vi "Programa_robot_final_3.vi"() -> ()   [LabVIEW 2019]
uses:
  <vilib>/Instr/_visa.llb/VISA Configure Serial Port (Instr).vi
  Global_STOP.vi
  <vilib>/regexp/Match Regular Expression.xnode
panel:
  in  "STOP TEST 3":bool
  in  "stop socket 4":bool
  in  "Abrir socket 2":bool
  in  "Cerrar socket 2":bool
  in  "Interruptor Error 2":bool
  in  "stop 4":bool
  in  "stop 3":bool
  in  "stop 2":bool
  in  "stop socket 3":bool
  out "Datos_QR":string
  in  "Interruptor Error":bool
  in  "Cerrar socket":bool
  in  "Abrir socket":bool
  out "Error_QR":bool
  out "return count":u32
  out "lectura puerto serie":u32
  out "dato escrito puerto serie":string
  out "OK, Fault 2":bool
  out "error out":errorcluster {"code" format="%f"}
  in  "STOP TEST 2":bool
  out "Datos_QR 2":string
  out "NUMERO ASICS TESTEADOS":i32
  out ".not. x?":bool
  in  "Config File":path=path "C:/Trabajo_Robot/Test Asic Javi_2021/Origen Socket SERVO_PCB_BUENO_v5 (muchos asics)/CONFIG/configuracion_robot_CTAV2022A.test"
  in  "SELECCION DE TEST":string(combo)
  in  "?":bool
  out "Boolean":bool
  in  "stop socket 2":bool
  out "Bytes at port 3":u32=1
  in  "IN y":string(combo)="00"
  in  "IN x":string(combo)="00"
  in  "NOK y":string(combo)="00"
  in  "NOK x":string(combo)="00"
  in  "OK y":string(combo)="00"
  in  "OK x":string(combo)="00"
  in  "Operator's name":string(combo)="Juan Rodríguez"
  in  "?":bool
  in  "Fichero de registro":path=path "C:/Trabajo_Robot/Pruebas/Pruebas.txt"
  in  "Path Out Report":path=path "C:/Trabajo_Robot/desde Marzo 2023/Pruebas_PC_APD/RESULT_TEST_C_LABP0/Test_33_ASIC_Referencia"
  in  "stop socket":bool
  out "Bytes at port 1":u32
  out "Iteraciones":i32
  out "Lectura buffer":string="1"
  in  "Delay (ms)":dbl=1.0 min=1.0 max=9.0 step=1.0
  out "Bytes at port 2":u32=1
  in  "Interruptor":bool=TRUE
  in  "stop":bool
  # "SI SE PRESIONA EL BOTON STOP PARA DETENER EL TEST,\nHAY QUE APAGAR Y VOLVER A ENCENDER EL ARDUINO"
  # "x: columna en cada bandeja \ny: fila en cada bandeja"
  # "Funcionamiento: en la primera iteración, el efector se desplaza desde el origen hasta la celda\nintroducida, hace una pausa, va a la posición del socket (0,0), hace otra pausa, va a la celda\nde salida y vuelve al origen. En las iteraciones siguientes hará lo mismo pero recorriendo las\nceldas de la bandeja sucesivamente. Que el desplazamiento se produzca hacia una celda de\nla bandeja OK o de la bandeja NOK depende de la salidad del programa de test de Asics."
types:
  T1 = enum16{"open", "replace", "create", "open or create", "replace or create", "replace or create with confirmation"}
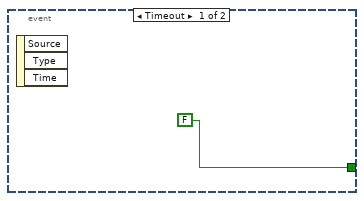
[diagram p2: hidden frame]
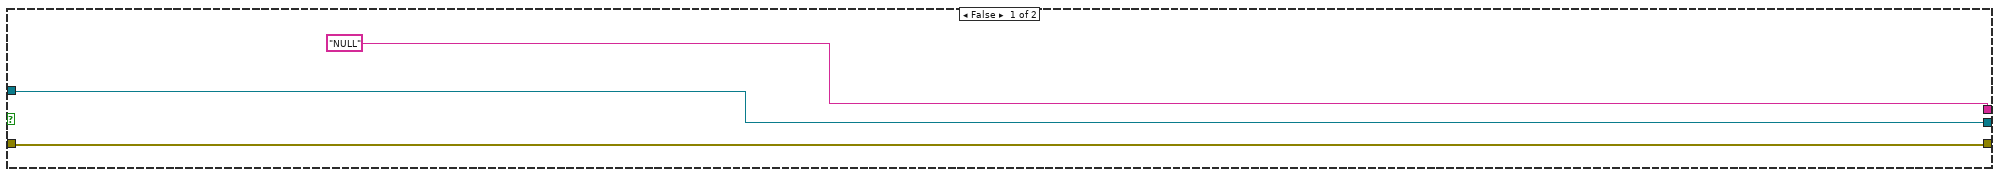
[diagram p5: hidden frame]
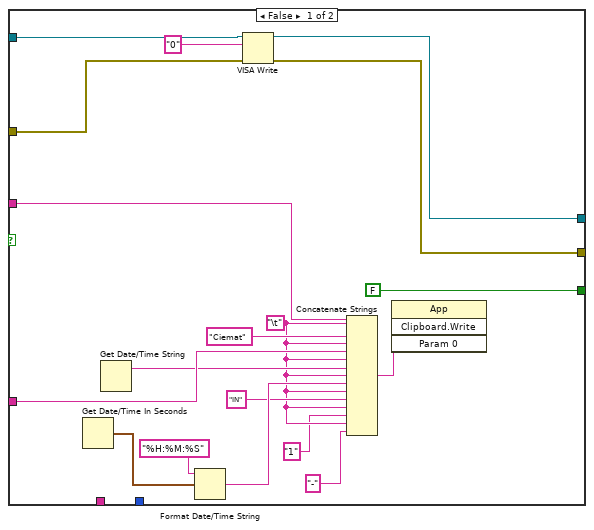
[diagram p7: hidden frame]
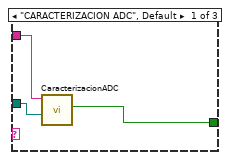
[diagram p8: hidden frame]
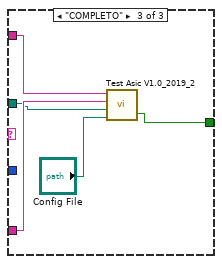
[diagram p9: hidden frame]
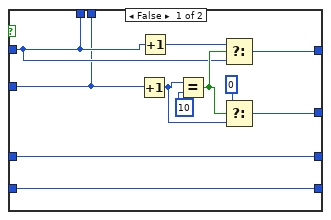
[diagram p11: hidden frame]
diagram:
  n1 = control-ref of="stop 2"() -> ()  [unwired: 1 out]
  n2 = control-ref of="stop 3"() -> ()  [unwired: 1 out]
  n3 = control-ref of="stop socket 3"() -> ()  [unwired: 1 out]
  n4 = control-ref of="Cerrar socket"() -> (w11:refnum<vi>)
  n5 = control-ref of="stop socket"() -> (w10:refnum<vi>)
  n6 = control-ref of="STOP TEST 2"() -> (w8:refnum<vi>)
  n7 = control-ref of="Abrir socket"() -> (w7:refnum<vi>)
  n8 = control-ref of="stop"() -> (w9:refnum<vi>)
  n9 = control-ref of="Interruptor Error"() -> (w12:refnum<vi>)
  n10 = property class="Bool (strict)"(reference=w8, "Visible"=FALSE) -> ()  [unwired: 1 in, 2 out]
  n11 = property class="Bool (strict)"(reference=w7, "Visible"=FALSE) -> ()  [unwired: 1 in, 2 out]
  n12 = property class="Bool (strict)"(reference=w12, "Visible"=FALSE) -> ()  [unwired: 1 in, 2 out]
  n13 = property class="Bool (strict)"(reference=w11, "Visible"=FALSE) -> ()  [unwired: 1 in, 2 out]
  n14 = property on="Boolean" class="Bool (strict)"("Visible"=FALSE) -> ()  [unwired: 2 in, 2 out]
  n15 = property class="Bool"(reference=w10, "Visible"=FALSE) -> ()  [unwired: 1 in, 2 out]
  n16 = property class="Bool"(reference=w9, "Visible"=FALSE) -> ()  [unwired: 1 in, 2 out]
  n17 = flat-sequence {
    tunnel: [w54] -> w18
    tunnel: ["Fichero de registro"] -> w17
    tunnel: ["SELECCION DE TEST"] -> w16
    tunnel: ["NOK y"] -> w33
    tunnel: ["NOK x"] -> w32
    tunnel: ["OK y"] -> w31
    tunnel: ["OK x"] -> w30
    tunnel: ["IN y"] -> w29
    tunnel: ["IN x"] -> w28
    tunnel: [w57] -> w27
    tunnel: [w58] -> w26
    tunnel: ["IN y"] -> w25
    tunnel: ["IN x"] -> w24
    tunnel: w17 -> [w56]
    frame #0 {
      n18 = while {
        stop <- "?" stop-if-true
        n19 = Not(x="?") -> (.not. x?=w50:bool)
        "Boolean" <- w50
        n20 = property on="Boolean" class="Bool (strict)"("Blinking"=w50) -> ()  [unwired: 2 in, 2 out]
      }
      n21 = global write "Global_STOP.vi" "stop"(FALSE ("stop")) -> ()
    }
    frame #1 {
      n22 = Not(x="?") -> (.not. x?=w54:bool)
      ".not. x?" <- w54
    }
    frame #2 {
      n23 = Open/Create/Replace File(file path (use dialog)=w56, operation (0:open)=T1."open", access (0:read/write)=enum16{"read/write", "read-only", "write-only"}."write-only") -> (refnum out=w69:refnum<file>, error out=w71:errorcluster)  [unwired: 3 in, 1 out]
      n24 = Set File Position(refnum=w69, from (0:start)=enum16{"start", "end", "current"}."end", error in=w71) -> (refnum out=w70:refnum<file>, error out=w72:errorcluster)  [unwired: 1 in]
      n25 = Write to Text File(file (use dialog)=w70, text="\r\n", error in=w72) -> (refnum out=w58:refnum<file>, error out=w57:errorcluster)  [unwired: 1 in, 1 out]
    }
  }
  n26 = Decimal String To Number(string=w25) -> (number=w23:i32)  [unwired: 2 in, 1 out]
  n27 = Decimal String To Number(string=w24) -> (number=w20:i32)  [unwired: 2 in, 1 out]
  n28 = Multiply(x=10, y=w23) -> (x*y=w21:i32)
  n29 = Decimal String To Number(string=w31) -> (number=w35:i32)  [unwired: 2 in, 1 out]
  n30 = Decimal String To Number(string=w30) -> (number=w34:i32)  [unwired: 2 in, 1 out]
  n31 = Decimal String To Number(string=w33) -> (number=w37:i32)  [unwired: 2 in, 1 out]
  n32 = Decimal String To Number(string=w32) -> (number=w36:i32)  [unwired: 2 in, 1 out]
  n33 = call-poly "VISA Configure Serial Port"("VISA resource name"=refnum<visa-resource-name> "COM9", "baud rate (9600)"=u32 9600, "data bits (8)"=u16 8) -> ("VISA resource name out"=w41:refnum<visa-resource-name>, "error out"=w44:errorcluster)  [unwired: 11 in]
  n34 = Add(x=w21, y=w20) -> (x+y=w19:i32)
  n35 = while {
    shift-right: [w82] -> w42
    shift-left: w44 -> [w123]
    tunnel: w41 -> [w121]
    tunnel: [w84] -> w43
    tunnel: w26 -> [w114]
    tunnel: [w113] -> w40
    tunnel: w27 -> [w112]
    tunnel: [w111] -> w39
    tunnel: w28 -> [w109]
    tunnel: w29 -> [w108]
    tunnel: w30 -> [w107]
    tunnel: w31 -> [w106]
    tunnel: w32 -> [w105]
    tunnel: w33 -> [w104]
    shift-right: [w97] -> _
    shift-left: w37 -> [w103]
    shift-right: [w99] -> _
    shift-left: w36 -> [w102]
    shift-right: [w96] -> _
    shift-left: w35 -> [w101]
    shift-right: [w98] -> _
    shift-left: w34 -> [w100]
    tunnel: w19 -> [w95]
    tunnel: w18 -> [w87]
    tunnel: w16 -> [w86]
    tunnel: [w80] -> w14
    i -> [w85]
    stop <- w80 stop-if-true
    n36 = flat-sequence {
      tunnel: w123 -> [w176]
      tunnel: w121 -> [w165]
      tunnel: [w167] -> w120
      tunnel: [w166] -> w119
      tunnel: w109 -> [w146]
      tunnel: w108 -> [w145]
      tunnel: w107 -> [w144]
      tunnel: w106 -> [w143]
      tunnel: w105 -> [w142]
      tunnel: w104 -> [w141]
      tunnel: w120 -> [w913]
      tunnel: w119 -> [w912]
      tunnel: [w911] -> w94
      tunnel: [w910] -> w92
      tunnel: [w909] -> _
      tunnel: w94 -> [w929]
      tunnel: [w927] -> w93
      tunnel: w92 -> [w928]
      tunnel: [w926] -> w91
      tunnel: w93 -> [w949]
      tunnel: w91 -> [w948]
      tunnel: w85 -> [w950]
      tunnel: [w946] -> w90
      tunnel: [w945] -> w89
      tunnel: [w944] -> w88
      tunnel: w85 -> [w1038]
      tunnel: [w1040] -> w117
      tunnel: [w1039] -> w116
      tunnel: [w1036] -> w110
      tunnel: w90 -> [w1035]
      tunnel: w89 -> [w1034]
      tunnel: w88 -> [w1033]
      tunnel: w87 -> [w1028]
      tunnel: w86 -> [w1031]
      tunnel: w85 -> [w1030]
      tunnel: [w1101] -> w115
      tunnel: [w1103] -> w118
      tunnel: w117 -> [w1102]
      tunnel: w116 -> [w1100]
      tunnel: w114 -> [w1107]
      tunnel: [w1106] -> w113
      tunnel: w112 -> [w1105]
      tunnel: [w1104] -> w111
      tunnel: w85 -> [w1097]
      tunnel: w110 -> [w1096]
      tunnel: w103 -> [w1092]
      tunnel: w102 -> [w1095]
      tunnel: w101 -> [w1094]
      tunnel: w100 -> [w1093]
      tunnel: [w1091] -> w97
      tunnel: [w1090] -> w99
      tunnel: [w1089] -> w96
      tunnel: [w1088] -> w98
      tunnel: w95 -> [w1087]
      tunnel: w85 -> [w1086]
      tunnel: [w1085] -> _
      frame #0 {
        n37 = for {
          N: 2 -> [_]
          shift-right: [w788] -> _
          shift-left: w146 -> [w793]
          shift-right: [w791] -> w162
          shift-left: w165 -> [w792]
          shift-right: [w789] -> w161
          shift-left: w176 -> [w790]
          n38 = xnode "Match Regular Expression"("input string"=w793, "regular expression"="-?\\d") -> ("whole match"=w787:string, "after match"=w788:string)  [unwired: 4 in, 3 out]
          n39 = VISA Write(VISA resource name=w792, write buffer=w787, error in (no error)=w790) -> (VISA resource name out=w791:refnum<visa-resource-name>, error out=w789:errorcluster)  [unwired: 1 out]
        }
        n40 = for {
          N: 2 -> [_]
          shift-right: [w666] -> _
          shift-left: w145 -> [w671]
          shift-right: [w669] -> w156
          shift-left: w162 -> [w670]
          shift-right: [w667] -> w155
          shift-left: w161 -> [w668]
          n41 = xnode "Match Regular Expression"("input string"=w671, "regular expression"="-?\\d") -> ("whole match"=w665:string, "after match"=w666:string)  [unwired: 4 in, 3 out]
          n42 = VISA Write(VISA resource name=w670, write buffer=w665, error in (no error)=w668) -> (VISA resource name out=w669:refnum<visa-resource-name>, error out=w667:errorcluster)  [unwired: 1 out]
        }
        n43 = for {
          N: 2 -> [_]
          shift-right: [w544] -> _
          shift-left: w144 -> [w549]
          shift-right: [w547] -> w158
          shift-left: w156 -> [w548]
          shift-right: [w545] -> w157
          shift-left: w155 -> [w546]
          n44 = xnode "Match Regular Expression"("input string"=w549, "regular expression"="-?\\d") -> ("whole match"=w543:string, "after match"=w544:string)  [unwired: 4 in, 3 out]
          n45 = VISA Write(VISA resource name=w548, write buffer=w543, error in (no error)=w546) -> (VISA resource name out=w547:refnum<visa-resource-name>, error out=w545:errorcluster)  [unwired: 1 out]
        }
        n46 = for {
          N: 2 -> [_]
          shift-right: [w422] -> _
          shift-left: w143 -> [w427]
          shift-right: [w425] -> w150
          shift-left: w158 -> [w426]
          shift-right: [w423] -> w149
          shift-left: w157 -> [w424]
          n47 = xnode "Match Regular Expression"("input string"=w427, "regular expression"="-?\\d") -> ("whole match"=w421:string, "after match"=w422:string)  [unwired: 4 in, 3 out]
          n48 = VISA Write(VISA resource name=w426, write buffer=w421, error in (no error)=w424) -> (VISA resource name out=w425:refnum<visa-resource-name>, error out=w423:errorcluster)  [unwired: 1 out]
        }
        n49 = for {
          N: 2 -> [_]
          shift-right: [w300] -> _
          shift-left: w142 -> [w305]
          shift-right: [w303] -> w152
          shift-left: w150 -> [w304]
          shift-right: [w301] -> w151
          shift-left: w149 -> [w302]
          n50 = xnode "Match Regular Expression"("input string"=w305, "regular expression"="-?\\d") -> ("whole match"=w299:string, "after match"=w300:string)  [unwired: 4 in, 3 out]
          n51 = VISA Write(VISA resource name=w304, write buffer=w299, error in (no error)=w302) -> (VISA resource name out=w303:refnum<visa-resource-name>, error out=w301:errorcluster)  [unwired: 1 out]
        }
        n52 = for {
          N: 2 -> [_]
          shift-right: [w178] -> _
          shift-left: w141 -> [w183]
          shift-right: [w181] -> w148
          shift-left: w152 -> [w182]
          shift-right: [w179] -> w147
          shift-left: w151 -> [w180]
          n53 = xnode "Match Regular Expression"("input string"=w183, "regular expression"="-?\\d") -> ("whole match"=w177:string, "after match"=w178:string)  [unwired: 4 in, 3 out]
          n54 = VISA Write(VISA resource name=w182, write buffer=w177, error in (no error)=w180) -> (VISA resource name out=w181:refnum<visa-resource-name>, error out=w179:errorcluster)  [unwired: 1 out]
        }
        n55 = Number To Decimal String(number="Delay (ms)") -> (decimal integer string=w170:string)  [unwired: 1 in]
        n56 = VISA Write(VISA resource name=w148, write buffer=w170, error in (no error)=w147) -> (VISA resource name out=w172:refnum<visa-resource-name>, error out=w171:errorcluster)  [unwired: 1 out]
        n57 = Select(t="1" ("write buffer"), s="Interruptor", f="0" ("write buffer")) -> (s? t:f=w168:string)
        n58 = VISA Write(VISA resource name=w172, write buffer=w168, error in (no error)=w171) -> (VISA resource name out=w167:refnum<visa-resource-name>, error out=w166:errorcluster)  [unwired: 1 out]
      }
      frame #1 {
        n59 = while {
          shift-right: [w919] -> w910
          shift-left: w912 -> [w924]
          tunnel: ["stop socket"] -> _
          shift-right: [w920] -> w911
          shift-left: w913 -> [w925]
          tunnel: ["stop socket"] -> w909
          stop <- w914 stop-if-true
          n60 = property class="Instr"(reference=w925, error in=w924) -> (reference out=w923:refnum<visa-resource-name>, error out=w922:errorcluster, "Bytes at Port"=w921:u32)
          "Bytes at port 1" <- w921
          n61 = VISA Read(VISA resource name=w923, byte count=w921, error in (no error)=w922) -> (VISA resource name out=w920:refnum<visa-resource-name>, read buffer=w918:string, error out=w919:errorcluster)  [unwired: 1 out]
          n62 = Equal?(x="2", y=w918) -> (x = y?=w916:bool)
          n63 = Or(x=w916, y="stop socket") -> (x .or. y?=w914:bool)
        }
      }
      frame #2 {
        n64 = while {
          shift-right: [w935] -> w926
          shift-left: w928 -> [w940]
          tunnel: ["stop socket 2"] -> _
          shift-right: [w936] -> w927
          shift-left: w929 -> [w941]
          tunnel: ["stop socket 2"] -> _
          stop <- w930 stop-if-true
          n65 = property class="Instr"(reference=w941, error in=w940) -> (reference out=w939:refnum<visa-resource-name>, error out=w938:errorcluster, "Bytes at Port"=w937:u32)
          "Bytes at port 3" <- w937
          n66 = VISA Read(VISA resource name=w939, byte count=w937, error in (no error)=w938) -> (VISA resource name out=w936:refnum<visa-resource-name>, read buffer=w934:string, error out=w935:errorcluster)  [unwired: 1 out]
          n67 = Equal?(x="3", y=w934) -> (x = y?=w932:bool)
          n68 = Or(x=w932, y="stop socket 2") -> (x .or. y?=w930:bool)
        }
      }
      frame #3 {
        # "Este bloque realiza la captura y lectura del QR"
        n69 = Greater?(x=w950, y=-1) -> (0:w947:bool)
        n70 = case shown="True" w947 {
          tunnel: [w954 w956] -> w944
          tunnel: w949 -> [w954 w958]
          tunnel: [w953 w957] -> w946
          tunnel: w948 -> [w953 w959]
          tunnel: ["NULL" ("Datos_QR") w955] -> w945
          frame False {
          }
          frame True {
            n71 = while {
              tunnel: [w973] -> w955
              tunnel: w958 -> [w971]
              tunnel: [w967] -> w956
              tunnel: [w966] -> w957
              tunnel: w959 -> [w961]
              stop <- w962 stop-if-true
              n72 = for {
                N: 10 -> [_]
                tunnel: [w1021] -> w973
                tunnel: [w1022] -> w962
                stop <- w1022 stop-if-true
                n73 = call "CapturaImagenyQR_subVI.vi"() -> ("Datos_QR"=w1021:string)  [unwired: 11 in]
                "Datos_QR" <- w1021
                n74 = Equal?(x=w1021, y="" ("Datos_QR")) -> (x = y?=w1023:bool)
                n75 = Not(x=w1023) -> (.not. x?=w1022:bool)
              }
              n76 = Select(t="1" ("write buffer"), s=w962, f="0" ("write buffer")) -> (s? t:f=w968:string)
              n77 = Not(x=w962) -> (.not. x?=→"Error_QR":bool)
              n78 = VISA Write(VISA resource name=w971, write buffer=w968, error in (no error)=w961) -> (VISA resource name out=w965:refnum<visa-resource-name>, error out=w964:errorcluster)  [unwired: 1 out]
              n79 = case shown="False" w962 {
                tunnel: w965 -> [w985 w1020]
                tunnel: w964 -> [w984 w1019]
                tunnel: [w983 w1020] -> w967
                tunnel: [w982 w1019] -> w966
                frame False {
                  n80 = flat-sequence {
                    tunnel: w985 -> [w989]
                    tunnel: [w988] -> w981
                    tunnel: [w987] -> w979
                    tunnel: w984 -> [w986]
                    tunnel: w981 -> [w1000]
                    tunnel: [w1000] -> w980
                    tunnel: w979 -> [w999]
                    tunnel: [w999] -> w978
                    tunnel: w980 -> [w1004]
                    tunnel: w978 -> [w1003]
                    tunnel: [w1002] -> w977
                    tunnel: [w1001] -> w975
                    tunnel: w977 -> [w1015]
                    tunnel: [w1015] -> w976
                    tunnel: w975 -> [w1014]
                    tunnel: [w1014] -> w974
                    tunnel: [w1016] -> w982
                    tunnel: [w1017] -> w983
                    tunnel: w976 -> [w1017]
                    tunnel: w974 -> [w1016]
                    frame #0 {
                      n81 = while {
                        tunnel: w989 -> [w997]
                        tunnel: [w992] -> w988
                        tunnel: [w991] -> w987
                        tunnel: w986 -> [w990]
                        stop <- "Abrir socket" stop-if-true
                        n82 = Select(t="2" ("write buffer"), s="Abrir socket", f="0" ("write buffer")) -> (s? t:f=w994:string)
                        n83 = VISA Write(VISA resource name=w997, write buffer=w994, error in (no error)=w990) -> (VISA resource name out=w992:refnum<visa-resource-name>, error out=w991:errorcluster)  [unwired: 1 out]
                      }
                    }
                    frame #1 {
                      n84 = Wait (ms)(milliseconds to wait=u32 1000) -> ()  [unwired: 1 out]
                    }
                    frame #2 {
                      n85 = while {
                        tunnel: w1004 -> [w1008]
                        tunnel: w1003 -> [w1007]
                        tunnel: [w1006] -> w1002
                        tunnel: [w1005] -> w1001
                        stop <- "Cerrar socket" stop-if-true
                        n86 = Select(t="3" ("write buffer"), s="Cerrar socket", f="0" ("write buffer")) -> (s? t:f=w1010:string)
                        n87 = VISA Write(VISA resource name=w1008, write buffer=w1010, error in (no error)=w1007) -> (VISA resource name out=w1006:refnum<visa-resource-name>, error out=w1005:errorcluster)  [unwired: 1 out]
                      }
                    }
                    frame #3 {
                      n88 = Wait (ms)(milliseconds to wait=u32 1000) -> ()  [unwired: 1 out]
                    }
                    frame #4 {
                      n89 = while {
                        stop <- "Interruptor Error" stop-if-true
                      }
                    }
                  }
                }
                frame True {
                }
              }
            }
            n90 = Wait (ms)(milliseconds to wait=u32 10000) -> ()  [unwired: 1 out]
          }
        }
        n91 = control-ref of="STOP TEST 2"() -> (w943:refnum<vi>)
        n92 = property class="Bool (strict)"(reference=w943, "Visible"=TRUE) -> ()  [unwired: 1 in, 2 out]
      }
      frame #4 {
        n93 = global read "Global_STOP.vi" "stop"() -> (w1027:bool)
        n94 = Greater?(x=w1038, y=-1) -> (0:w1029:bool)
        n95 = Not(x=w1027) -> (.not. x?=w1026:bool)
        n96 = Compound Arithmetic op=AND(w1029, w1028, w1026) -> (w1025:bool)
        n97 = case shown="True" w1025 {
          tunnel: w1033 -> [w1056 w1063]
          tunnel: w1035 -> [w1055 w1062]
          tunnel: [w1054 w1061] -> w1040
          tunnel: [w1053 w1060] -> w1039
          tunnel: w1034 -> [w1049 w1070]
          tunnel: [FALSE ("Boolean") w1068] -> w1036
          tunnel: "Operator's name" -> [w1047 w1067]
          tunnel: w1031 -> [_ w1066]
          tunnel: w1030 -> [_ w1065]
          frame False {
            w1043 = "\t"
            n98 = Get Date/Time In Seconds() -> (seconds since 1Jan1904=w1051:timestamp)
            n99 = Get Date/Time String() -> (date string=w1046:string)  [unwired: 3 in, 1 out]
            n100 = Format Date/Time String(time format string (%c)="%H:%M:%S", seconds (now)=w1051) -> (date/time string=w1045:string)  [unwired: 1 in]
            n101 = VISA Write(VISA resource name=w1056, write buffer="0", error in (no error)=w1055) -> (VISA resource name out=w1054:refnum<visa-resource-name>, error out=w1053:errorcluster)  [unwired: 1 out]
            n102 = Concatenate Strings(w1049, w1043, "Ciemat", w1043, w1047, w1043, w1046, w1043, w1045, w1043, "IN", w1043, "1", w1043, "-") -> (w1052:string)
            n103 = invoke class="App" method="Clipboard.Write"("Param 0"=w1052) -> ()  [unwired: 3 in, 4 out]
          }
          frame True {
            # "Test de Asics"
            n104 = case shown="\"SUMAS 3 CANALES\"" w1066 {
              tunnel: w1070 -> [w1075 w1077 w1084]
              tunnel: "Path Out Report" -> [w1074 w1079 w1082]
              tunnel: [w1073 w1078 w1080] -> w1068
              tunnel: w1067 -> [_ _ w1083]
              tunnel: w1065 -> [_ w1076 _]
              frame "CARACTERIZACION ADC", Default {
                n105 = call "CaracterizacionADC.vi"("QR code"=w1075, "Path Out Report"=w1074) -> ("OK/NOK"=w1073:bool)  [unwired: 7 in]
              }
              frame "SUMAS 3 CANALES" {
                n106 = call "Test_Sumadores_Javi.vi"("QR"=w1077, "Path"=w1079, "NUMERO DE PASADA DE TEST"=w1076) -> ("Boolean"=w1078:bool)  [unwired: 8 in]
                "NUMERO ASICS TESTEADOS" <- w1076
              }
              frame "COMPLETO" {
                n107 = call "Test Asic V1.0_2019_2.vi"("Config File"="Config File", "Path Out Report"=w1082, "Operator's Name"=w1083, "ASIC'S Number"=w1084) -> ("OK, Fault 2"=w1080:bool)  [unwired: 1 in]
              }
            }
            "OK, Fault 2" <- w1068
            n108 = Select(t="1" ("write buffer"), s=w1068, f="0" ("write buffer")) -> (s? t:f=w1064:string)
            "dato escrito puerto serie" <- w1064
            n109 = VISA Write(VISA resource name=w1063, write buffer=w1064, error in (no error)=w1062) -> (VISA resource name out=w1061:refnum<visa-resource-name>, return count=→"return count":u32, error out=w1060:errorcluster)
          }
        }
      }
      frame #5 {
        n110 = Greater?(x=w1097, y=-1) -> (0:w1098:bool)
        n111 = case shown="True" w1098 {
          tunnel: w1107 -> [w1113 w1146]
          tunnel: [w1113 w1145] -> w1106
          tunnel: w1105 -> [w1112 w1144]
          tunnel: [w1112 w1143] -> w1104
          tunnel: [w1115 w1142] -> w1103
          tunnel: w1102 -> [w1115 w1142]
          tunnel: [w1114 w1141] -> w1101
          tunnel: w1100 -> [w1114 w1141]
          tunnel: w1096 -> [_ w1139]
          tunnel: w1092 -> [w1111 w1138]
          tunnel: w1095 -> [w1110 w1137]
          tunnel: w1094 -> [w1109 w1136]
          tunnel: w1093 -> [w1108 w1135]
          tunnel: [w1111 w1134] -> w1091
          tunnel: [w1110 w1133] -> w1090
          tunnel: [w1109 w1132] -> w1089
          tunnel: [w1108 w1131] -> w1088
          frame False {
          }
          frame True {
            w1118 = "\t"
            # "Registro de datos en fichero"
            n112 = invoke class="App" method="Clipboard.Read"() -> ("Read Clipbrd"=w1140:string)  [unwired: 3 in, 2 out]
            n113 = case shown="True" w1139 {
              tunnel: w1138 -> [w1149 w1162]
              tunnel: w1137 -> [w1148 w1161]
              tunnel: w1136 -> [w1151 w1159]
              tunnel: w1135 -> [w1150 w1160]
              tunnel: [w1153 w1162] -> w1134
              tunnel: [w1152 w1161] -> w1133
              tunnel: [w1151 w1164] -> w1132
              tunnel: [w1150 w1163] -> w1131
              tunnel: [w1149 w1159] -> w1130
              tunnel: [w1148 w1160] -> w1129
              frame False {
                n114 = Increment(x=w1148) -> (x+1=w1157:i32)
                n115 = Increment(x=w1149) -> (x+1=w1154:i32)
                n116 = Equal?(x=w1157, y=10) -> (x = y?=w1155:bool)
                n117 = Select(t=w1154, s=w1155, f=w1149) -> (s? t:f=w1153:i32)
                n118 = Select(t=0, s=w1155, f=w1157) -> (s? t:f=w1152:i32)
              }
              frame True {
                n119 = Increment(x=w1160) -> (x+1=w1168:i32)
                n120 = Increment(x=w1159) -> (x+1=w1165:i32)
                n121 = Equal?(x=w1168, y=10) -> (x = y?=w1166:bool)
                n122 = Select(t=w1165, s=w1166, f=w1159) -> (s? t:f=w1164:i32)
                n123 = Select(t=0, s=w1166, f=w1168) -> (s? t:f=w1163:i32)
              }
            }
            n124 = Write to Text File(file (use dialog)=w1146, text=w1140, error in=w1144) -> (refnum out=w1127:refnum<file>, error out=w1128:errorcluster)  [unwired: 1 in, 1 out]
            n125 = Number To Decimal String(number=w1130) -> (decimal integer string=w1117:string)  [unwired: 1 in]
            n126 = Number To Decimal String(number=w1129) -> (decimal integer string=w1116:string)  [unwired: 1 in]
            n127 = Write to Text File(file (use dialog)=w1127, text=w1118, error in=w1128) -> (refnum out=w1125:refnum<file>, error out=w1126:errorcluster)  [unwired: 1 in, 1 out]
            n128 = Write to Text File(file (use dialog)=w1125, text=w1117, error in=w1126) -> (refnum out=w1122:refnum<file>, error out=w1121:errorcluster)  [unwired: 1 in, 1 out]
            n129 = Write to Text File(file (use dialog)=w1122, text=w1118, error in=w1121) -> (refnum out=w1120:refnum<file>, error out=w1119:errorcluster)  [unwired: 1 in, 1 out]
            n130 = Write to Text File(file (use dialog)=w1120, text=w1116, error in=w1119) -> (refnum out=w1124:refnum<file>, error out=w1123:errorcluster)  [unwired: 1 in, 1 out]
            n131 = Write to Text File(file (use dialog)=w1124, text="\r\n", error in=w1123) -> (refnum out=w1145:refnum<file>, error out=w1143:errorcluster)  [unwired: 1 in, 1 out]
          }
        }
        n132 = Add(x=w1087, y=w1086) -> (x+y=w1085:i32)
      }
    }
    n133 = while {
      shift-right: [w1177] -> w76
      shift-left: w115 -> [w1183]
      tunnel: ["stop"] -> _
      shift-right: [w1178] -> w84
      shift-left: w118 -> [w1184]
      tunnel: [w1173] -> w122
      stop <- w1171 stop-if-true
      # "1"
      # "Mientras se ejecuta este bucle (la espera a que\nArduino termine una iteración), cambiamos los\ndatos de los controladores."
      n134 = property class="Instr"(reference=w1184, error in=w1183) -> (reference out=w1181:refnum<visa-resource-name>, error out=w1180:errorcluster, "Bytes at Port"=w1179:u32)
      "Bytes at port 2" <- w1179
      n135 = VISA Read(VISA resource name=w1181, byte count=w1179, error in (no error)=w1180) -> (VISA resource name out=w1178:refnum<visa-resource-name>, read buffer=w1173:string, return count=w1176:u32, error out=w1177:errorcluster)
      "lectura puerto serie" <- w1176
      n136 = Greater Or Equal?(x=w1176, y=u32 1) -> (x >= y?=w1174:bool)
      n137 = global read "Global_STOP.vi" "stop"() -> (w1170:bool)
      n138 = Or(x=w1174, y="stop") -> (x .or. y?=w1172:bool)
      n139 = Compound Arithmetic op=OR(w1172, w1170) -> (w1171:bool)
    }
    "Lectura buffer" <- w122
    n140 = flat-sequence {
      tunnel: w76 -> [w125]
      tunnel: [w125] -> w75
      tunnel: [w124] -> w73
      frame #0 {
        n141 = global read "Global_STOP.vi" "stop"() -> (w124:bool)
      }
    }
    n142 = case shown="False" w73 {
      selector: w73 -> [_ w135]
      tunnel: [w129 _] -> w81
      tunnel: [w126 w135] -> w77
      tunnel: w75 -> [w127 w134]
      tunnel: [w127 w134] -> w74
      frame False {
        n143 = for {
          N: 3 -> [_]
          tunnel: [w132] -> _
          tunnel: [w130] -> w129
          tunnel: [w130] -> w126
          stop <- w130 stop-if-true
          n144 = call "CapturaImagenyQR_subVI.vi"() -> ("Datos_QR"=w132:string)  [unwired: 11 in]
          "Datos_QR 2" <- w132
          n145 = Equal?(x=w132, y="" ("Datos_QR")) -> (x = y?=w131:bool)
          n146 = Not(x=w131) -> (.not. x?=w130:bool)
        }
      }
      frame True {
      }
    }
    n147 = flat-sequence {
      tunnel: [w138] -> w80
      tunnel: w77 -> [w136]
      frame #0 {
        n148 = global read "Global_STOP.vi" "stop"() -> (w137:bool)
        n149 = Or(x=w136, y=w137) -> (x .or. y?=w138:bool)
      }
    }
    n150 = Boolean To (0,1)(Boolean=w81) -> (0, 1=w79:i16)
    n151 = call <vilib>:"Error Cluster From Error Code.vi"("error in (no error)"=w74, "error message (\"\")"="El asic no se ha colocado en la\n    bandeja de salida,se ha quedado\nen el socket posiblemente por una\nmala succión de la ventosa.\nPresione STOP\n" ("error message (\"\")"), "error code (0)"=w79) -> ("error out"=w78:errorcluster)  [unwired: 6 in]
    n152 = call <vilib>:"Simple Error Handler.vi"("error in (no error)"=w78) -> ("error out"=w82:errorcluster)  [unwired: 4 in, 4 out]
    n153 = case shown="True" w81 {
      selector: w81 -> [w139 w140]
      tunnel: [w139 w140] -> _
      frame False {
      }
      frame True {
        n154 = call "Send Email2"() -> ()  [unwired: 11 in, 1 out]
      }
    }
    "Iteraciones" <- w85
  }
  n155 = flat-sequence {
    frame #0 {
      n156 = local write "STOP TEST 2"(FALSE ("STOP TEST 2")) -> ()
    }
    frame #1 {
      n157 = while {
        stop <- w1186 stop-if-true
        n158 = event shown="[1] \"STOP TEST 2\": Value Change" {
          selector: _ -> [_ _]
          dyn-events: _ -> [_ _]
          timeout: _ -> [_ _]
          tunnel: [FALSE "STOP TEST 2"] -> w1186
          event Timeout {
            n159 = event-data() -> ()  [unwired: 1 in, 3 out]
          }
          event "STOP TEST 2": Value Change {
            n160 = event-data() -> ()  [unwired: 1 in, 6 out]
            n161 = global write "Global_STOP.vi" "stop"("STOP TEST 2") -> ()
            n162 = Wait (ms)(milliseconds to wait=u32 100) -> ()  [unwired: 1 out]
          }
        }
      }
    }
  }
  n163 = Close File(refnum=w40, error in=w39) -> (error out=w38:errorcluster)  [unwired: 1 out]
  n164 = Not(x=w14) -> (.not. x?=w15:bool)
  n165 = call <vilib>:"Simple Error Handler.vi"("error in (no error)"=w38) -> ()  [unwired: 4 in, 5 out]
  n166 = global write "Global_STOP.vi" "stop"(w15) -> ()
  n167 = VISA Close(VISA resource name=w43, error in (no error)=w42) -> (error out=→"error out":errorcluster)
